vi "SEA_9811_count_Chn_Rx_words.vi"(7 "channel #":i32, 8 "error in (no error)":errorcluster, 11 "SEA9811_RT_data in":T1) -> (0 "error out":errorcluster, 3 "SEA9811_RT_data out":T1, 5 "received words":u32)   [LabVIEW 2012]
doc: "gets this channels Rx word count"
uses:
  Typdefs/SEA9811_RT_data_cluster.ctl
  Typdefs/FPGA ref.ctl
  Typdefs/channel.ctl
  Typdefs/received word.ctl
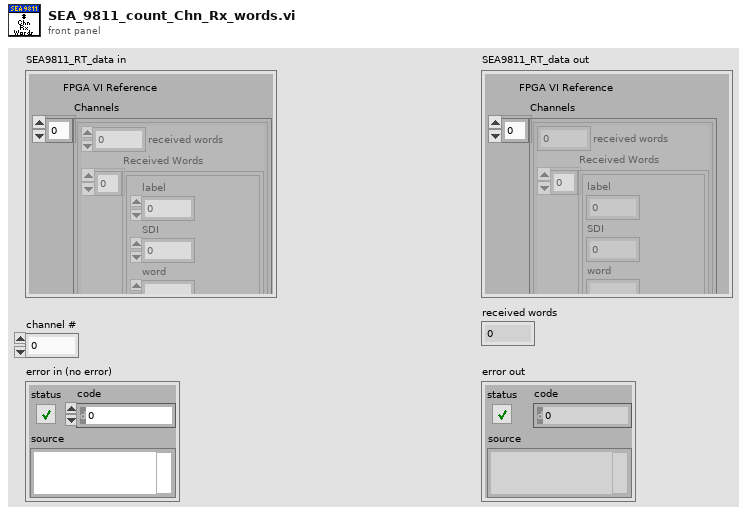
[diagram p1: front panel]
types:
  T1 = typedef "SEA9811_RT_data_cluster.ctl" = cluster{"FPGA VI Reference":T2, "Channels":T3[]}
  T2 = typedef "FPGA ref.ctl" = refnum<k20>
  T3 = typedef "channel.ctl" = cluster{"received words":u32, "Received Words":T4[]}
  T4 = typedef "received word.ctl" = cluster{"label":u8, "SDI":u8, "word":u32, "timestamp":dbl}
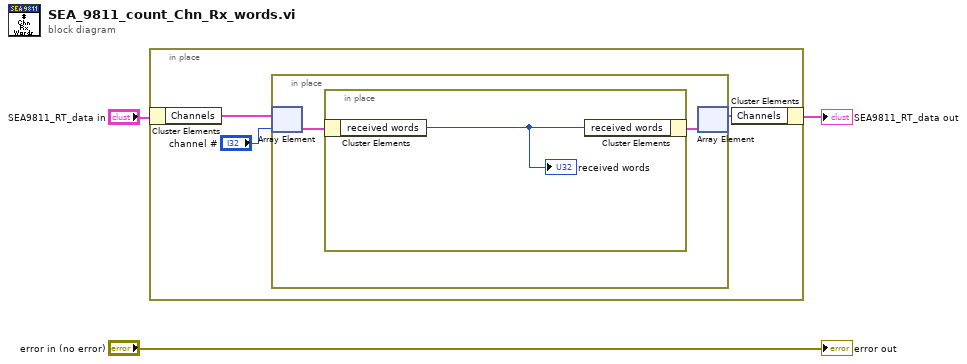
[diagram p0: block diagram]
diagram:
  n1 = in-place {
    n2 = in-place-cluster #1("SEA9811_RT_data in") -> ("Channels"=w6:T3[])
    n3 = in-place {
      n4 = in-place-array #2(w6, "channel #") -> (w8:T3)
      n5 = in-place {
        n6 = in-place-cluster #3(w8) -> ("received words"=w9:u32)
        "received words" <- w9
        n7 = in-place-cluster #3("received words"=w9) -> (w7:T3)
      }
      n8 = in-place-array #2(w7) -> (w4:T3[])  [unwired: 1 out]
    }
    n9 = in-place-cluster #1("Channels"=w4) -> (→"SEA9811_RT_data out":T1)
  }
  "error out" <- "error in (no error)"
